vi "Test Kinematics.vi"() -> ()   [LabVIEW 2017]
uses:
  <vilib>/Platform/TimedLoop/XDataNode/timing_clust.ctl
  <vilib>/Platform/TimedLoop/XDataNode/nitl_modes.ctl
  <vilib>/Platform/TimedLoop/XDataNode/wakeup.ctl
  <vilib>/Analysis/baseanly.llb/A x Vector.vi
  <vilib>/Analysis/_algsub.llb/Vector Norm.vi
  <vilib>/Analysis/_algsub.llb/Real Vector Norm.vi
  <vilib>/Analysis/baseanly.llb/Outer Product.vi
  <vilib>/Analysis/baseanly.llb/Real Outer Product.vi
  <vilib>/robotics/Kinematics/Create Lie Group Matrix.vi
  <vilib>/Analysis/7linalg.llb/Create Special Matrix.vi
  <vilib>/Analysis/7linalg.llb/Create Special Real Matrix.vi
  <vilib>/Analysis/Matrix/Numeric/Multiply/Multiply.vi
  <vilib>/Analysis/Matrix/Numeric/Multiply/Multiply - RM,R.vi
  <vilib>/Analysis/Matrix/Numeric/Multiply/Multiply - R,RM.vi
  <vilib>/Analysis/Matrix/Numeric/Add/Add.vi
  <vilib>/Analysis/Matrix/Numeric/Add/Add - RM,RM.vi
  <vilib>/platform/TimedLoop/XDataNode/XDataNode.xnode
  <vilib>/robotics/Kinematics/NI_Kinematics.lvlib
  <vilib>/Analysis/NI_AALBase.lvlib
  <vilib>/Platform/TimedLoop/XDataNode/XDNodeRunTimeDep.lvlib
panel:
  in  "theta0":dbl[](array[numeric])=[0.0, 0.0, 0.0] format="%#_15g"
  in  "Kd":dbl=0.01 format="%#_13g"
  in  "Kp":dbl=10.0 format="%#_13g"
  out "thetac":dbl[](array[numeric])=[-0.9695710575831353, -0.9695710575831351, -0.9695710575831353] format="%#_15g"
  out "v3c":dbl[](array[numeric])=[0.003384567298342642, -0.6787074301172594, 0.7344009592912673]
  out "v1c":dbl[](array[numeric])=[0.5860856101152999, 0.3422849249434341, 0.7344009039838837]
  out "v2c":dbl[](array[numeric])=[-0.589470227845441, 0.3364226533042573, 0.7344008774692956]
  out "beta2":dbl=0.7460127831658564
  out "v30":dbl[](array[numeric])=[-0.5877852522924729, 0.33935797363675174, 0.7344008870614411]
  out "v10":dbl[](array[numeric])=[0.0, -0.6787159472735029, 0.7344008870614411]
  out "v20":dbl[](array[numeric])=[0.5877852522924731, 0.3393579736367513, 0.7344008870614411]
  in  "phi":dbl(knob) scale=-3.14..3.14
  out "dt":dbl=0.001
  in  "Period":i64=1
  out "v2d":dbl[](array[numeric])=[-0.5932269079867079, 0.32975319971745287, 0.7344008870614411]
  out "v1d":dbl[](array[numeric])=[0.5821881019278716, 0.3488729726662565, 0.7344008870614411]
  out "v3d":dbl[](array[numeric])=[0.011038806058836004, -0.6786261723837091, 0.7344008870614411]
  out "thetad":dbl[](array[numeric])=[-0.9708927453046908, -0.9708927453046906, -0.9708927453046908] format="%#_15g"
  out "message":string="No Error"
  out "error?":bool
  in  "stop":bool
  out "beta1":dbl=0.9553166181245093
  out "gamma2":dbl=1.2566370614359172
  out "gamma1":dbl=1.5707963267948966
  out "alpha2":dbl=1.5707963267948966
  out "alpha1":dbl=1.5707963267948966
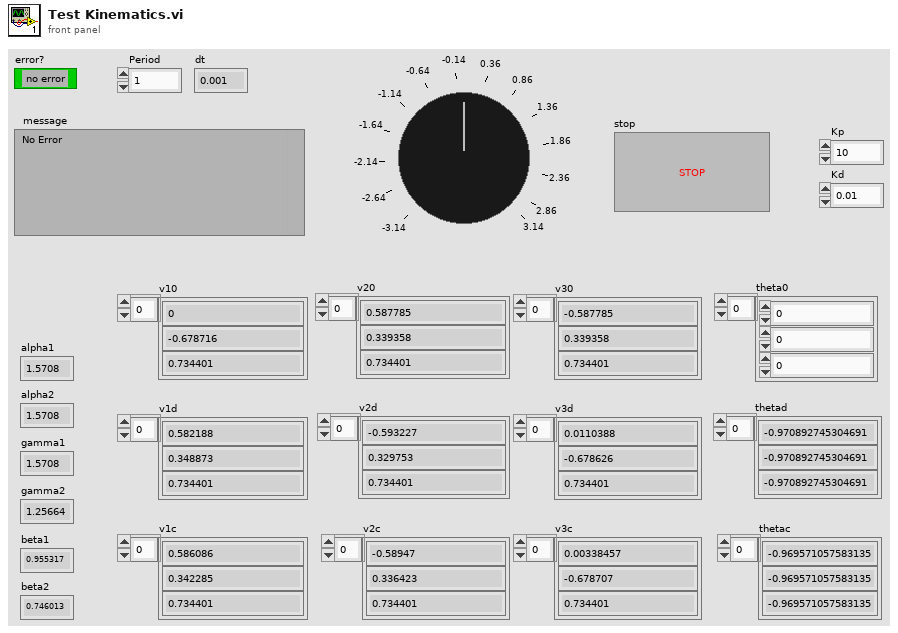
[diagram p1: front panel]
types:
  T1 = typedef "XDNodeRunTimeDep.lvlib/timing_clust.ctl" = cluster{"Expected End [f-1]":u64, "Actual End [f-1]":u64, "Finished Late? [f-1]":bool, "Expected End [i-1]":u64, "Actual End [i-1]":u64, "Finished Late? [i-1]":bool, "Expected Start [i]":u64, "Actual Start [i]":u64, "Expected Start [f]":u64, "Actual Start [f]":u64, "Source Name":string, "Structure Name":string, "Period":i64, "Deadline":i64, "Offset":i64, "Start":i64, "Priority":i32, "Timeout":i32, "Mode":T2, "Wakeup Reason":T3, "Error":errorcluster, "Source Type":string, "Secondary Source Type":string, "Global End Time":u64, "Global Start Time":u64, "Frame Duration":u64, "Iteration Duration":u64, "Assigned CPU":i32, "I/O Scan Engine Mode":u32}
  T2 = typedef "XDNodeRunTimeDep.lvlib/nitl_modes.ctl" = enum32{"No Change", "Process missed periods, maintain original phase", "Discard missed periods, maintain original phase", "Process missed periods, ignore original phase", "Discard missed periods, ignore original phase"}
  T3 = typedef "XDNodeRunTimeDep.lvlib/wakeup.ctl" = enum32{"Normal", "Aborted", "Asynchronous wakeup", "Timing source error", "Timed loop error", "Timeout"}
  T4 = typedef "NI_Matrix.lvlib/RealMatrix.ctl" = dbl[][]
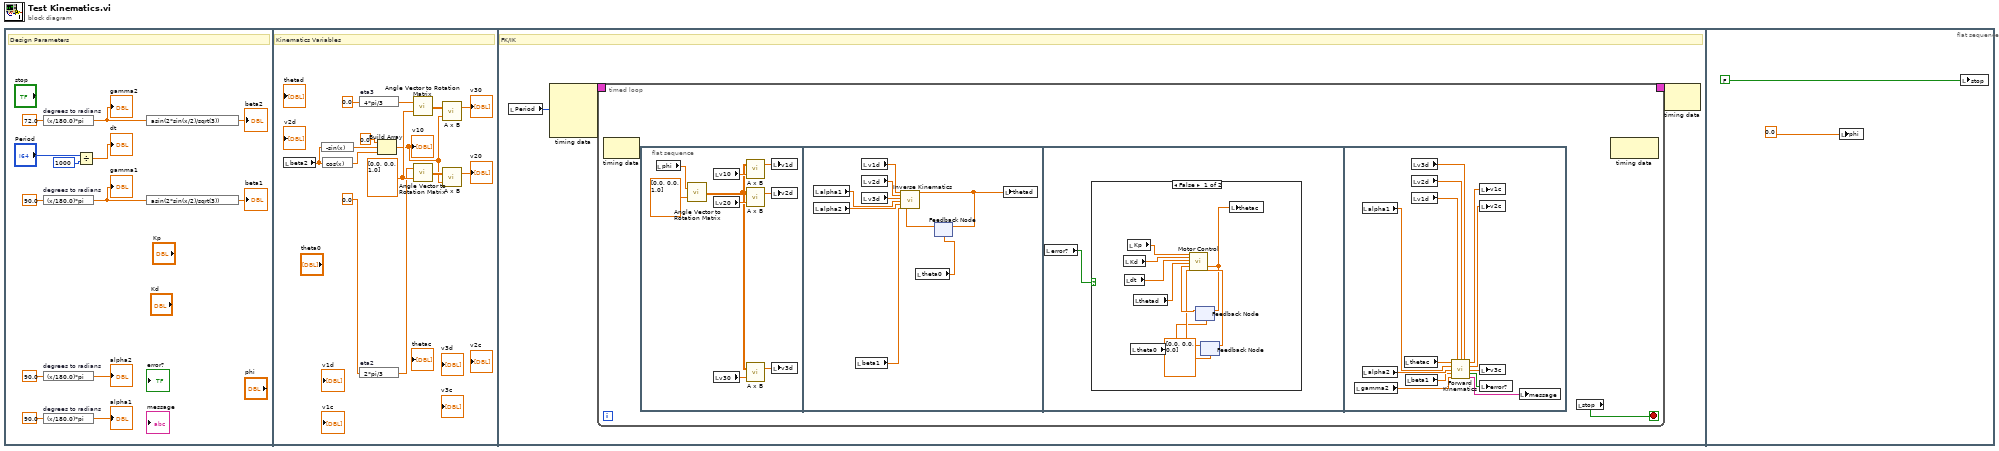
[diagram p0: block diagram]
diagram:
  n1 = flat-sequence {
    frame #0 {
      # "Design Parameters"
      n2 = expression code="(x/180.0)*pi" "degrees to radians"(72.0 ("gamma2")) -> (w5:dbl)
      "gamma2" <- w5
      n3 = expression code="(x/180.0)*pi" "degrees to radians"(90.0 ("gamma1")) -> (w7:dbl)
      "gamma1" <- w7
      n4 = expression code="(x/180.0)*pi" "degrees to radians"(90.0 ("alpha2")) -> (→"alpha2":dbl)
      n5 = expression code="(x/180.0)*pi" "degrees to radians"(90.0 ("alpha1")) -> (→"alpha1":dbl)
      n6 = Divide(x="Period", y=i64 1000) -> (x/y=→"dt":dbl)
      n7 = expression code="asin(2*sin(x/2)/sqrt(3))"(w5) -> (→"beta2":dbl)
      n8 = expression code="asin(2*sin(x/2)/sqrt(3))"(w7) -> (→"beta1":dbl)
    }
    frame #1 {
      w24 = dbl[] [0.0, 0.0, 1.0] ("vector")
      # "Kinematics Variables"
      n9 = local read "beta2"() -> (w14:dbl)
      n10 = expression code="-sin(x)"(w14) -> (w26:dbl)
      n11 = expression code="cos(x)"(w14) -> (w25:dbl)
      n12 = expression code="4*pi/3" "eta3"(0.0) -> (w22:dbl)
      n13 = expression code="2*pi/3" "eta2"(0.0) -> (w23:dbl)
      n14 = Build Array(0.0 ("element"), w26, w25) -> (w17:dbl[])
      "v10" <- w17
      n15 = call <vilib>:"Angle Vector to Rotation Matrix.vi"("vector"=w24, "angle"=w22) -> ("rotation matrix"=w20:T4)
      n16 = call <vilib>:"Angle Vector to Rotation Matrix.vi"("vector"=w24, "angle"=w23) -> ("rotation matrix"=w21:T4)
      n17 = call-poly <vilib>:"A x B.vi"("Vector"=w17, "A"=w20) -> ("A x Vector"=→"v30":dbl[])  [unwired: 1 out]
      n18 = call-poly <vilib>:"A x B.vi"("Vector"=w17, "A"=w21) -> ("A x Vector"=→"v20":dbl[])  [unwired: 1 out]
    }
    frame #2 {
      # "FK/IK"
      n19 = local read "Period"() -> (w28:i64)
      n20 = node-c288(w28) -> (w30:T1)  [unwired: 3 in]
      n21 = timed-loop {
        timing: w30 -> [_]
        timing-out: [_] -> w29
        stop <- w31 stop-if-true
        n22 = node-c288() -> ()  [unwired: 1 in, 1 out]
        n23 = flat-sequence {
          frame #0 {
            n24 = local read "phi"() -> (w39:dbl)
            n25 = call <vilib>:"Angle Vector to Rotation Matrix.vi"("vector"=dbl[] [0.0, 0.0, 1.0], "angle"=w39) -> ("rotation matrix"=w35:T4)
            n26 = local read "v10"() -> (w38:dbl[])
            n27 = local read "v20"() -> (w37:dbl[])
            n28 = local read "v30"() -> (w36:dbl[])
            n29 = call-poly <vilib>:"A x B.vi"("Vector"=w38, "A"=w35) -> ("A x Vector"=w34:dbl[])  [unwired: 1 out]
            n30 = call-poly <vilib>:"A x B.vi"("Vector"=w37, "A"=w35) -> ("A x Vector"=w33:dbl[])  [unwired: 1 out]
            n31 = call-poly <vilib>:"A x B.vi"("Vector"=w36, "A"=w35) -> ("A x Vector"=w32:dbl[])  [unwired: 1 out]
            n32 = local write "v1d"(w34) -> ()
            n33 = local write "v2d"(w33) -> ()
            n34 = local write "v3d"(w32) -> ()
          }
          frame #1 {
            n35 = local read "alpha1"() -> (w46:dbl)
            n36 = local read "alpha2"() -> (w45:dbl)
            n37 = local read "beta1"() -> (w44:dbl)
            n38 = local read "v1d"() -> (w49:dbl[])
            n39 = local read "v2d"() -> (w48:dbl[])
            n40 = local read "v3d"() -> (w47:dbl[])
            n41 = local read "theta0"() -> (w42:dbl[])
            n42 = feedback #1(w42) -> (w41:dbl[])
            n43 = call "Inverse Kinematics.vi"("v1"=w49, "v2"=w48, "v3"=w47, "alpha1"=w46, "alpha2"=w45, "beta1"=w44, "theta"=w41) -> ("theta'"=w43:dbl[])  [unwired: 12 in]
            n44 = feedback-in #1(w43) -> ()
            n45 = local write "thetad"(w43) -> ()
          }
          frame #2 {
            n46 = local read "error?"() -> (w50:bool)
            n47 = case shown="False" w50 {
              frame False {
                n48 = local read "Kd"() -> (w59:dbl)
                n49 = local read "dt"() -> (w58:dbl)
                n50 = local read "Kp"() -> (w60:dbl)
                n51 = local read "theta0"() -> (w53:dbl[])
                n52 = local read "thetad"() -> (w57:dbl[])
                n53 = feedback #2(w53) -> (w56:dbl[])
                n54 = feedback #3(dbl[] [0.0, 0.0, 0.0] ("e'")) -> (w54:dbl[])
                n55 = call "Motor Control.vi"("Kp"=w60, "Kd"=w59, "dt"=w58, "thetad"=w57, "thetac"=w56, "e"=w54) -> ("thetac'"=w51:dbl[], "e'"=w55:dbl[])  [unwired: 12 in]
                n56 = feedback-in #2(w51) -> ()
                n57 = feedback-in #3(w55) -> ()
                n58 = local write "thetac"(w51) -> ()
              }
              frame True {
              }
            }
          }
          frame #3 {
            n59 = local read "gamma2"() -> (w66:dbl)
            n60 = local read "alpha1"() -> (w69:dbl)
            n61 = local read "alpha2"() -> (w68:dbl)
            n62 = local read "thetac"() -> (w70:dbl[])
            n63 = local read "beta1"() -> (w67:dbl)
            n64 = local read "v3d"() -> (w73:dbl[])
            n65 = local read "v2d"() -> (w71:dbl[])
            n66 = local read "v1d"() -> (w72:dbl[])
            n67 = call "Forward Kinematics.vi"("theta"=w70, "v1"=w72, "v2"=w71, "v3"=w73, "alpha1"=w69, "alpha2"=w68, "beta1"=w67, "gamma2"=w66) -> ("v1'"=w65:dbl[], "v2'"=w64:dbl[], "v3'"=w63:dbl[], "error?"=w61:bool, "message"=w62:string)  [unwired: 3 in]
            n68 = local write "v1c"(w65) -> ()
            n69 = local write "v2c"(w64) -> ()
            n70 = local write "v3c"(w63) -> ()
            n71 = local write "error?"(w61) -> ()
            n72 = local write "message"(w62) -> ()
          }
        }
        n73 = local read "stop"() -> (w31:bool)
        n74 = node-c288() -> ()  [unwired: 1 in, 1 out]
      }
      n75 = node-c288(w29) -> ()  [unwired: 1 out]
    }
    frame #3 {
      n76 = local write "phi"(0.0 ("phi")) -> ()
      n77 = local write "stop"(FALSE ("stop")) -> ()
    }
  }
